vi "CSM - Module Status.vi"(8 "Error in":errorcluster caption="Error in (no error)", 11 "CSM Name":string) -> (0 "Error out":errorcluster, 1 "#Instance":i32, 2 "Mode":T1=enum."Stand Alone", 3 "CSM Name(dup)":string, 4 "#msg to be processed":i32)   [LabVIEW 2020, in "Communicable State Machine.lvlib"]
doc: "Get the CSM+ Module Status\n\n<b>Inputs:</b>\n - <b>CSM Name</b>: CSM module name.\n - <b>Error in</b>: Error cluster\n\n<b>Outputs:</b>\n - <b>Mode</b>: Return the mode of CSM Module. It might be \"Stand-alone\", \"CSM\" or \"Action Worker\".\n - <b>#As Worker</b>: Number of the workers if module in \"Action Worker\" mode.\n - <b>#msg to be processed</b>: The number of message in CSM Message Queue.\n - <b>CSM Name(dup)</b>: Return <b>CSM Name</b>\n - <b>Error out</b>: Error cluster"
uses:
  Communicable State Machine.lvlib
  _CSM_MODE.ctl
  _CSMOFGVOPER.ctl
  Priority Queue.lvclass/Priority Queue.ctl
  Priority Queue.lvclass
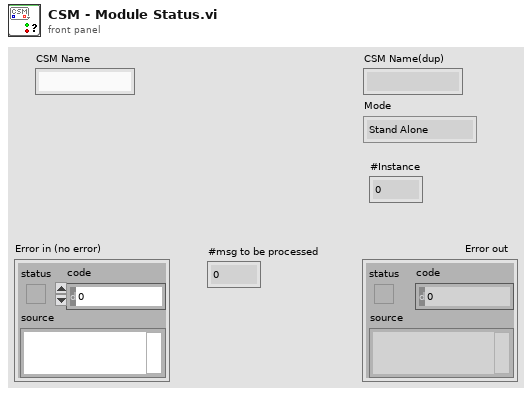
[diagram p1: front panel]
types:
  T1 = typedef "Communicable State Machine.lvlib/_CSM_MODE.ctl" = enum16{"Not Exist", "Stand Alone", "CSM", "Worker Agent", "Worker", "Chain", "Chain Node"}
  T2 = typedef "Communicable State Machine.lvlib/_CSMOFGVOPER.ctl" = enum16{"Create If not Exist", "Get By Name", "List", "Check If Name Exists", "Release", "Module Status", "Create Status Event Handler", "Destroy Status Event Handler"}
  T3 = typedef "Communicable State Machine.lvlib/_CSMObj.ctl" = cluster{"Requested Name":string, "Module Name":string, "Mode":T1, "Queue":refnum<class "Priority Queue.lvclass">, "CSM-Data":refnum<data-value>, "User Event":refnum<user-event>, "Status Change Event":refnum<user-event>, "Allowed Messages":string[], "Mode-Data":refnum<data-value>, "Group Name":string, "Exit Event":refnum<user-event>}
  T4 = typedef "Communicable State Machine.lvlib/_CSMObj-ModeData.ctl" = cluster{"Share Count":i32, "Messages of Chain Nodes":cluster{"Module Name":string, "Allowed Messages":string[]}[], "Chain Message Mapping Map":variant}
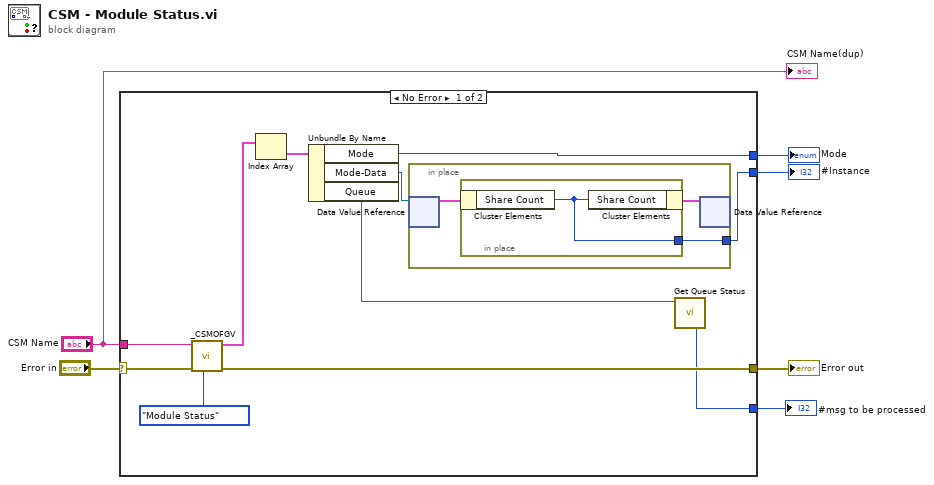
[diagram p0: block diagram]
diagram:
  n1 = case shown="No Error" "Error in" {
    selector: "Error in" -> [w17 w22]
    tunnel: [w16 w22] -> w5
    tunnel: [w12 _] -> w4
    tunnel: [w10 _] -> w3
    tunnel: "CSM Name" -> [w9 _]
    tunnel: [w7 _] -> w1
    frame No Error {
      n2 = call "_CSMOFGV.vi"("Operation"=_CSMOFGVOPER."Module Status", "Error in"=w17, "Name(\"\" to use uuid) in"=w9) -> ("Error out"=w16:errorcluster, "Array"=w14:T3[])  [unwired: 6 in, 1 out]
      n3 = Index Array(array=w14) -> (element=w13:T3)  [unwired: 1 in]
      n4 = Unbundle By Name(w13) -> ("Mode"=w12:T1, "Mode-Data"=w8:refnum<data-value>, "Queue"=w11:refnum<class "Priority Queue.lvclass">)
      n5 = in-place {
        in-place-border: [w18] -> w7
        n6 = in-place-dvr #1(w8) -> (w20:T4)  [unwired: 1 out]
        n7 = in-place {
          in-place-border: [w21] -> w18
          n8 = in-place-cluster #2(w20) -> ("Share Count"=w21:i32)
          n9 = in-place-cluster #2("Share Count"=w21) -> (w19:T4)
        }
        n10 = in-place-dvr #1(w19) -> ()  [unwired: 2 out]
      }
      n11 = call "Get Queue Status.vi"("Priority Queue in"=w11) -> ("# elements in queue"=w10:i32)  [unwired: 6 in, 4 out]
    }
    frame Error {
    }
  }
  "Error out" <- w5
  "Mode" <- w4
  "#Instance" <- w1
  "#msg to be processed" <- w3
  "CSM Name(dup)" <- "CSM Name"
